vi "dfd_TF to SOS.vi"(8 "UP?":bool, 10 "denominator":dbl[](array[numeric]) format="%.2f", 11 "numerator":dbl[](array[numeric]) format="%.2f") -> (2 "SOS reverse coefficients":dbl[](array[numeric]) format="%.2f", 3 "SOS forward coefficients":dbl[](array[numeric]) format="%.2f")   [LabVIEW 2017, in "NI_DigFilterLicensed.lvlib"]
uses:
  <vilib>/addons/Digital Filter Design/NI_DigFilterLicensed.lvlib
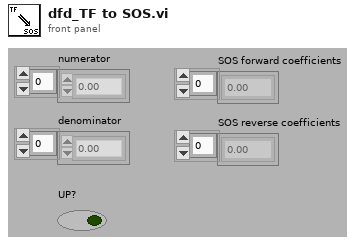
[diagram p1: front panel]
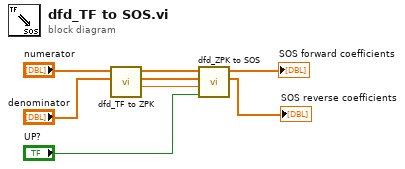
[diagram p0: block diagram]
diagram:
  n1 = call <vilib>:"dfd_TF to ZPK.vi"("denominator"="denominator", "numerator"="numerator") -> ("gain"=w3:dbl, "poles"=w2:cdb[], "zeros"=w6:cdb[])  [unwired: 7 out]
  n2 = call <vilib>:"dfd_ZPK to SOS.vi"("UP?"="UP?", "gain"=w3, "poles"=w2, "zeros"=w6) -> ("SOS reverse coefficients"=→"SOS reverse coefficients":dbl[], "SOS forward coefficients"=→"SOS forward coefficients":dbl[])  [unwired: 6 out]
